vi "S2C_Initialize.vi"(8 "Error In":errorcluster, 10 "MenuRef":refnum<k9>, 11 "This VI":refnum<vi>) -> (0 "Error Out":errorcluster)   [LabVIEW 2015]
doc: "Aquires front panel references, initializes the front panel, read all setting from the settings file, and reads all configurations from the config file."
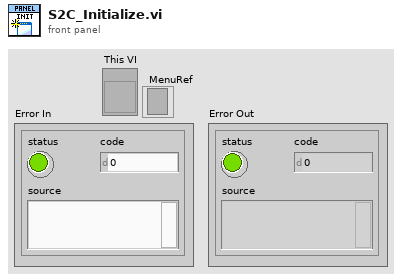
[diagram p1: front panel]
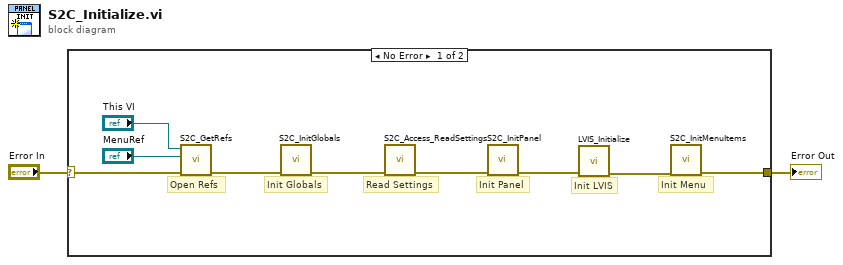
[diagram p0: block diagram]
diagram:
  n1 = case shown="No Error" "Error In" {
    selector: "Error In" -> [w11 w12]
    tunnel: [w3 w12] -> w2
    frame No Error {
      # "Read Settings"
      # "Init Menu"
      # "Init LVIS"
      # "Open Refs"
      # "Init Panel"
      # "Init Globals"
      n2 = call "S2C_GetRefs.vi"("Error In"=w11, "MenuRef"="MenuRef", "VI Ref"="This VI") -> ("Error Out"=w9:errorcluster)  [unwired: 8 in]
      n3 = call "S2C_InitGlobals.vi"("Error In"=w9) -> ("Error Out"=w7:errorcluster)  [unwired: 10 in]
      n4 = call "S2C_Access_ReadSettings.vi"("Error In"=w7) -> ("Error Out"=w6:errorcluster)  [unwired: 10 in]
      n5 = call "S2C_InitPanel.vi"("Error In"=w6) -> ("Error Out"=w5:errorcluster)  [unwired: 10 in]
      n6 = call "LVIS_Initialize.vi"("Error In"=w5) -> ("Error Out"=w4:errorcluster)  [unwired: 9 in, 1 out]
      n7 = call "S2C_InitMenuItems.vi"("Error In"=w4) -> ("Error Out"=w3:errorcluster)  [unwired: 10 in]
    }
    frame Error {
    }
  }
  "Error Out" <- w2
